vi "Check SSIS Import Table.vi"(8 "error IN":errorcluster, 11 "Site":string) -> (0 "error OUT":errorcluster, 2 "max expt rec":string="0", 3 "max shot id rec":string="0")   [LabVIEW 2015]
uses:
  <vilib>/addons/database/Connection.llb/DB Tools Open Connec (Path).vi
  <vilib>/addons/database/Connection.llb/Conn Execute.vi
  <vilib>/addons/database/Recordset.llb/Rec Destroy - Connection.vi
  <vilib>/addons/database/NI_Database_API.lvlib
panel:
  out "App.Dir":path
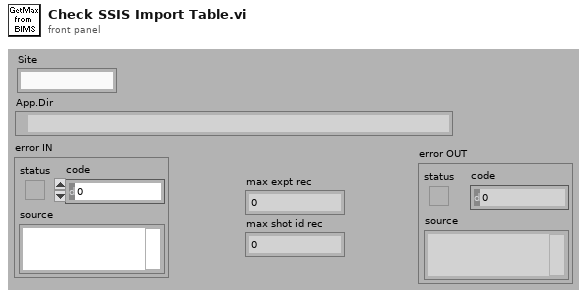
[diagram p1: front panel]
types:
  T1 = typedef "NI_Database_API.lvlib/Conn ObjectReference.ctl" = refnum<k1>
  T2 = typedef "NI_Database_API.lvlib/Rec ObjectReference.ctl" = refnum<k1>
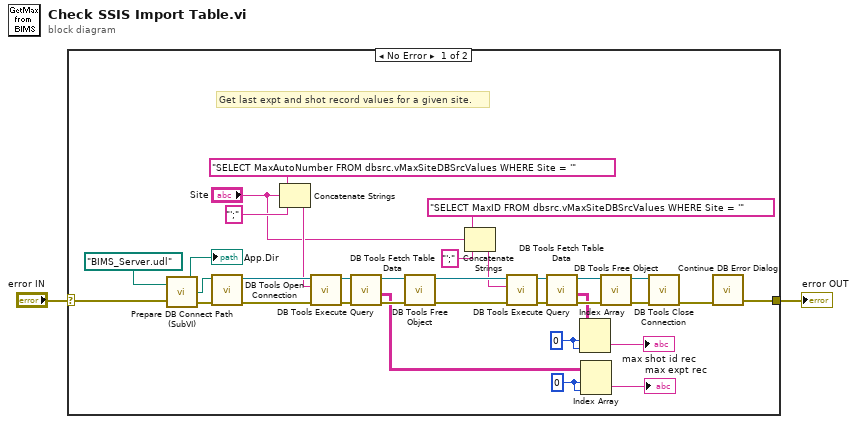
[diagram p0: block diagram]
diagram:
  n1 = case shown="No Error" "error IN" {
    selector: "error IN" -> [w7 w37]
    tunnel: [w15 w37] -> w2
    frame No Error {
      w19 = 0 ("index (row)")
      w22 = 0 ("index (row)")
      # "Get last expt and shot record values for a given site."
      n2 = call "Prepare DB Connect Path (SubVI).vi"("connectString"=path "BIMS_Server.udl", "error in"=w7) -> ("App.Dir"=→"App.Dir":path, "appended path"=w4:path, "error out"=w6:errorcluster)
      n3 = call-poly <vilib>:"DB Tools Open Connection.vi"("error in (no error)"=w6, "connection information"=w4) -> ("error out"=w34:errorcluster, "connection reference"=w33:T1)  [unwired: 3 in, 3 out]
      n4 = Concatenate Strings("SELECT MaxAutoNumber FROM dbsrc.vMaxSiteDBSrcValues WHERE Site = '" ("message"), "Site", "';" ("message")) -> (w12:string)
      n5 = call-poly <vilib>:"DB Tools Execute Query.vi"("error in (no error)"=w34, "SQL query"=w12, "connection reference"=w33) -> ("error out"=w35:errorcluster, "recordset reference"=w32:T2)  [unwired: 1 in, 4 out]
      n6 = call <vilib>:"DB Tools Fetch Table Data.vi"("error in (no error)"=w35, "recordset reference"=w32) -> ("error out"=w36:errorcluster, "recordset data"=w23:string[][], "recordset reference out"=w31:T2)  [unwired: 3 out]
      n7 = call-poly <vilib>:"DB Tools Free Object.vi"("error in (no error)"=w36, "recordset reference"=w31) -> ("error out"=w16:errorcluster, "connection reference"=w17:T1)  [unwired: 8 out]
      n8 = Concatenate Strings("SELECT MaxID FROM dbsrc.vMaxSiteDBSrcValues WHERE Site = '" ("message"), "Site", "';" ("message")) -> (w8:string)
      n9 = call-poly <vilib>:"DB Tools Execute Query.vi"("error in (no error)"=w16, "SQL query"=w8, "connection reference"=w17) -> ("error out"=w25:errorcluster, "recordset reference"=w26:T2)  [unwired: 1 in, 4 out]
      n10 = call <vilib>:"DB Tools Fetch Table Data.vi"("error in (no error)"=w25, "recordset reference"=w26) -> ("error out"=w24:errorcluster, "recordset data"=w18:string[][], "recordset reference out"=w27:T2)  [unwired: 3 out]
      n11 = Index Array(array=w18, index (row)=w19, index (col)=w19) -> (element=→"max shot id rec":string)
      n12 = Index Array(array=w23, index (row)=w22, index (col)=w22) -> (element=→"max expt rec":string)
      n13 = call-poly <vilib>:"DB Tools Free Object.vi"("error in (no error)"=w24, "recordset reference"=w27) -> ("error out"=w29:errorcluster, "connection reference"=w30:T1)  [unwired: 8 out]
      n14 = call <vilib>:"DB Tools Close Connection.vi"("error in (no error)"=w29, "connection reference"=w30) -> ("error out"=w28:errorcluster)  [unwired: 5 out]
      n15 = call "Continue DB Error Dialog.vi"("error in (no error)"=w28) -> ("error out"=w15:errorcluster)  [unwired: 3 in, 2 out]
    }
    frame Error {
    }
  }
  "error OUT" <- w2
